vi "waitMotorStop.vi"(8 "error in (no error)":errorcluster, 11 "VISA Refnum in":refnum<visa-resource-name>) -> (0 "error out":errorcluster, 3 "VISA Refnum out":refnum<visa-resource-name>)   [LabVIEW 2014]
doc: "Newport Motion Controler\nThis sub VI Wait Motor Stop\n\nAndré Romero - 2020\nandretec@ifsc.usp.br"
uses:
  <userlib>/Newport ESP301/Newport ESP301.lvlib
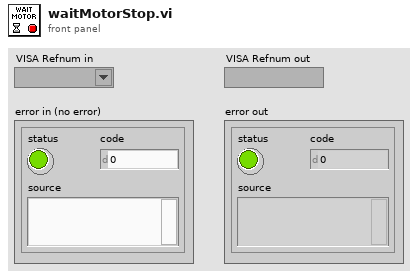
[diagram p1: front panel]
types:
  T1 = cluster{"Axis1 moving":bool, "Axis2 moving":bool, "Axis3 moving":bool, "Axis4 moving":bool, "Motor Power of at least one axis":bool, "Reserved":bool, "Reserved":bool, "Reserved":bool, "Axis5 moving 2":bool, "Axis6 moving 2":bool, "Reserved":bool, "Reserved":bool, "Motor Power of at least one axis":bool, "Reserved":bool, "Reserved":bool, "Reserved":bool}
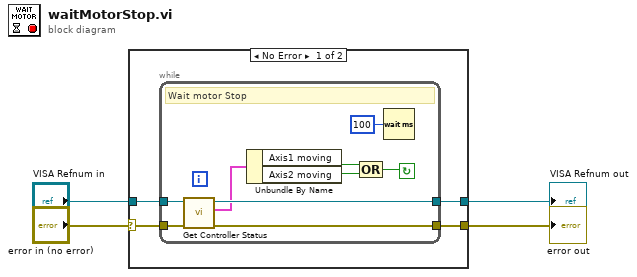
[diagram p0: block diagram]
diagram:
  n1 = case shown="No Error" "error in (no error)" {
    selector: "error in (no error)" -> [w8 w18]
    tunnel: "VISA Refnum in" -> [w7 w19]
    tunnel: [w6 w19] -> w3
    tunnel: [w5 w18] -> w4
    frame No Error {
      n2 = while {
        tunnel: [w16] -> w6
        tunnel: w8 -> [w17]
        tunnel: [w15] -> w5
        tunnel: w7 -> [w9]
        stop <- w11 continue-if-true
        # "Wait motor Stop"
        n3 = call <userlib>:"Get Controller Status.vi"("error in (no error)"=w17, "VISA resource name"=w9) -> ("error out"=w15:errorcluster, "Controller Status"=w14:T1, "VISA resource name out"=w16:refnum<visa-resource-name>)  [unwired: 2 in, 1 out]
        n4 = Unbundle By Name(w14) -> ("Axis1 moving"=w13:bool, "Axis2 moving"=w12:bool)
        n5 = Compound Arithmetic op=OR(w13, w12) -> (w11:bool)
        n6 = Wait (ms)(milliseconds to wait=u32 100) -> ()  [unwired: 1 out]
      }
    }
    frame Error {
    }
  }
  "error out" <- w4
  "VISA Refnum out" <- w3
